vi "test Read U32.vi"(8 "error in (no error)":errorcluster, 11 "TestCase in":refnum<class "Buffer Tests.lvclass">) -> (0 "error out":errorcluster, 3 "TestCase out":refnum<class "Buffer Tests.lvclass">)   [LabVIEW 2019, in "Buffer Tests.lvclass"]
uses:
  Buffer Tests.lvclass
  <vilib>/NI/Memory Manager/Classes/Pointer/Pointer.lvclass/Pointer.ctl
  <vilib>/NI/Memory Manager/Classes/Pointer/Get Internal.vi
  <vilib>/NI/Memory Manager/Classes/Pointer/Errors.vi
  <vilib>/NI/Memory Manager/Classes/Pointer/Zone.vi
  <vilib>/NI/Memory Manager/Classes/Pointer/Set Address.vi
  <vilib>/NI/Memory Manager/Classes/Pointer/Set Size.vi
  <vilib>/NI/Memory Manager/Classes/Pointer/Set Internal.vi
  <vilib>/NI/Memory Manager/Classes/Pointer/Get Address.vi
  <vilib>/NI/Memory Manager/Classes/Pointer/Check Null Pointer.vi
  <vilib>/NI/Memory Manager/Classes/Pointer/Create Error.vi
  <vilib>/NI/Memory Manager/Classes/Pointer/Null Pointer.vi
  <vilib>/NI/Memory Manager/Classes/Pointer/Is Null.vi
  <vilib>/NI/Memory Manager/VIs/New Error Cluster.vi
  <vilib>/NI/Memory Manager/VIs/New Error Cluster (512B).vi
  <vilib>/NI/Memory Manager/VIs/Set Error Status.vi
  <vilib>/NI/Memory Manager/VIs/Set Error Code.vi
  <vilib>/NI/Memory Manager/VIs/Set Error Source.vi
  <vilib>/NI/Memory Manager/Constants/Constants.vi
  <vilib>/NI/Memory Manager/Constants/Library Name.vi
  <vilib>/NI/Memory Manager/Classes/Pointer/Pointer Error Info.vi
  <vilib>/NI/Memory Manager/VIs/Write String to Source.vi
  <vilib>/NI/Memory Manager/Constants/Pointer Class Name.vi
  Classes/Buffer/Buffer.lvclass
  C:/Program Files (x86)/National Instruments/LabVIEW 2019/vi.lib/NI/Memory Manager/Classes/Pointer/Pointer.lvclass
  Classes/Buffer/Read Buffer 0D U32.vi
  <vilib>/addons/_JKI Toolkits/VI Tester/TestCase.llb/TestCase.lvclass
  <vilib>/NI/Memory Manager/Classes/Pointer/Pointer.lvclass
  C:/Program Files (x86)/National Instruments/LabVIEW 2019/vi.lib/addons/_JKI Toolkits/VI Tester/TestCase.llb/TestCase.lvclass
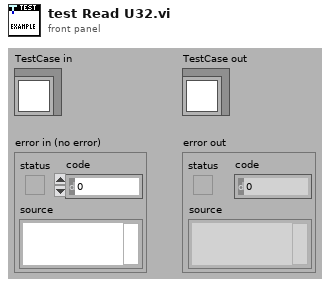
[diagram p1: front panel]
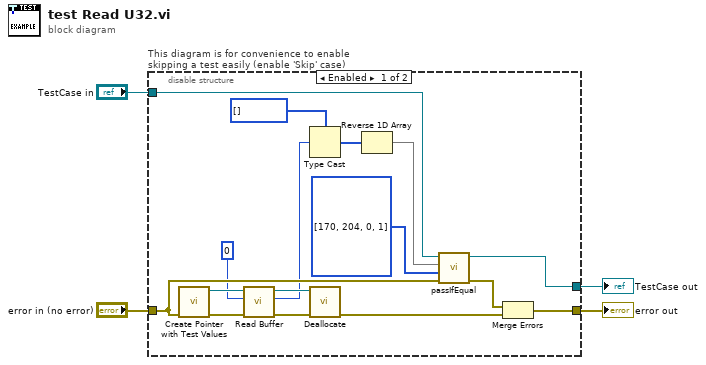
[diagram p0: block diagram]
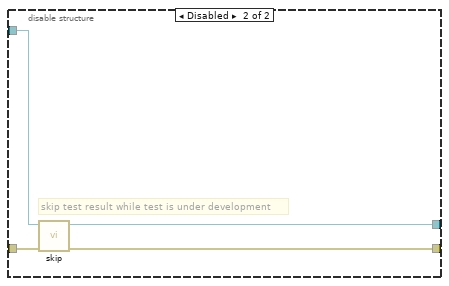
[diagram p2: hidden frame]
diagram:
  n1 = disable-structure "This diagram is for convenience to enable skipping a test easily (enable 'Skip' case)" shown="Enabled" {
    disable-tunnel: "TestCase in" -> [w12 w24]
    disable-tunnel: [w15 w22] -> w1
    disable-tunnel: [w10 w23] -> w2
    disable-tunnel: "error in (no error)" -> [w11 w21]
    frame Enabled {
      n2 = call "Create Pointer with Test Values.vi"("error in (no error)"=w11) -> ("error out"=w8:errorcluster, "Buffer out"=w6:refnum<class "Buffer.lvclass">)  [unwired: 9 in]
      n3 = call-poly "Read Buffer.vi"("error in (no error)"=w8, "dst value in"=u32 0, "Buffer in"=w6) -> ("error out"=w19:errorcluster, "dst value out"=w9:u32, "Buffer out"=w20:refnum<class "Buffer.lvclass">)  [unwired: 5 in, 1 out]
      n4 = Type Cast(type=u8[] [] ("buffer in"), x=w9) -> (*(type *) &x=w18:u8[])
      n5 = call <vilib>:"Deallocate.vi"("error in (no error)"=w19, "Pointer"=w20) -> ("error out"=w7:errorcluster)  [unwired: 8 in, 1 out]
      n6 = Reverse 1D Array(array=w18) -> (reversed array=w13:u8[])
      n7 = call-dynamic "passIfEqual.vi"("error in (no error)"=w11, "y"=u8[] [170, 204, 0, 1] ("subarray 2"), "x"=w13, "TestCase in"=w12) -> ("error out"=w16:errorcluster, "TestCase out"=w15:refnum<class "Buffer Tests.lvclass">)  [unwired: 6 in]
      n8 = Merge Errors(w16, w7) -> (w10:errorcluster)
    }
    frame Disabled {
      # "skip test result while test is under development"
      n9 = call <vilib>:"skip.vi"("error in (no error)"=w21, "TestCase in"=w24) -> ("error out"=w23:errorcluster, "TestCase out"=w22:refnum<class "Buffer Tests.lvclass">)  [unwired: 8 in]
    }
  }
  "error out" <- w2
  "TestCase out" <- w1
